vi "Write Cource OutputOffset.vi"(8 "error in (no error)":errorcluster, 10 "Cource OutputOffset":bool=TRUE, 11 "BME_DG_G08_Chnl in":refnum<class "BME_DG_G08_Chnl.lvclass">) -> (0 "error out":errorcluster, 3 "BME_DG_G08_Chnl out":refnum<class "BME_DG_G08_Chnl.lvclass">)   [LabVIEW 2009, in "POLARIS BME DG.lvlib" / "BME_DG_G08_Chnl.lvclass"]
uses:
  BME_DG_G08_Chnl.lvclass
  BME_DG_G08_Chnl.lvclass/BME_DG_G08_Chnl.ctl
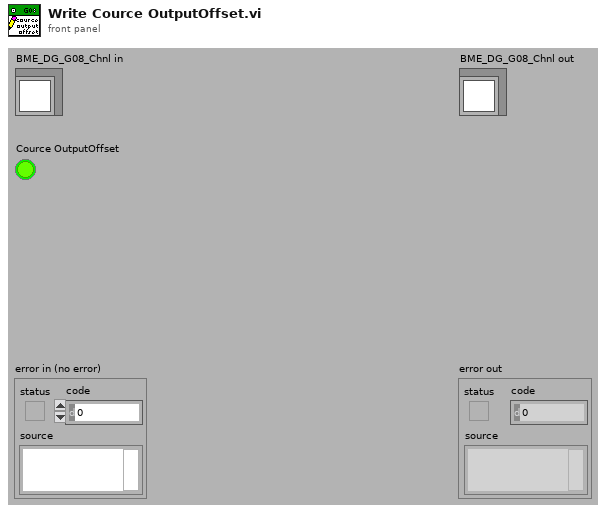
[diagram p1: front panel]
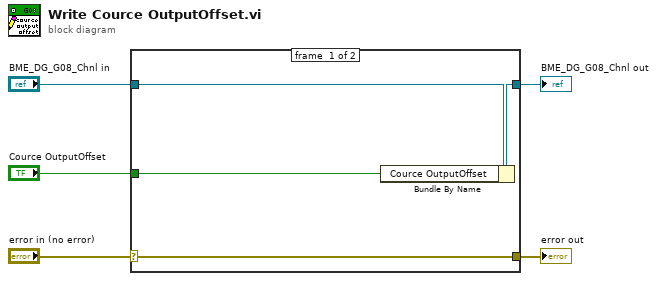
[diagram p0: block diagram]
diagram:
  n1 = case shown="No Error" "error in (no error)" {
    selector: "error in (no error)" -> [w9 w10]
    tunnel: [w9 w10] -> w4
    tunnel: [w7 w11] -> w2
    tunnel: "BME_DG_G08_Chnl in" -> [w8 w11]
    tunnel: "Cource OutputOffset" -> [w6 _]
    frame #0 {
      n2 = Bundle By Name(cluster=w8, "Cource OutputOffset"=w6) -> (w7:refnum<class "BME_DG_G08_Chnl.lvclass">)
    }
    frame #1 {
    }
  }
  "error out" <- w4
  "BME_DG_G08_Chnl out" <- w2
